vi "TARGET.vi"() -> ()   [LabVIEW 2018]
uses:
  <vilib>/Platform/TimedLoop/XDataNode/timing_clust.ctl
  <vilib>/Platform/TimedLoop/XDataNode/nitl_modes.ctl
  <vilib>/Platform/TimedLoop/XDataNode/wakeup.ctl
  <vilib>/rvi/eio/common/nirviEmuTemplateMethod_errors.vi
  <vilib>/rvi/Emulation/niFpgaGetClockAttributes.vi
  <vilib>/rvi/Emulation/niFpgaSctlEmulationGetInTimedLoop.vi
  <vilib>/rvi/Emulation/niFpgaEmulationReportErrorSimple.vi
  <vilib>/rvi/Emulation/niFpgaProcessEmulError.vi
  <vilib>/rvi/Emulation/niFpgaCriticalErrorInLSC.vi
  <vilib>/rvi/DataTransferAndStorage/Container/Common/niFpgaContainerGetUniqueNameForEmu.vi
  <vilib>/rvi/Memory/Memory_Emulation/niFpgaMemoryFastEmulationDramWriteAndRequestData.vi
  <vilib>/rvi/Memory/Memory_Emulation/niFpgaMemoryEmulationDramWriteAndRequestData.vi
  <vilib>/rvi/Memory/Memory_Emulation/niFpgaMemoryEmulationDramWriteAndRequestDataApplyByteEnables.vi
  <vilib>/rvi/interface/RandomDataEmulation/niFpgaRandomDataHandleErrors.vi
  <vilib>/eio/EIONode/EIONode.xnode
  <vilib>/Platform/TimedLoop/XDataNode/XDataNode.xnode
  <vilib>/rvi/DataTransferAndStorage/Container/XNode/niFpgaContainer.xnode
  <vilib>/rvi/Memory/Memory_Emulation/niFpgaMemoryEmulationDramRetrieveData.vi
  <vilib>/rvi/interface/RandomDataEmulation/nirviRandomDataFpgaReadWriteTemplate.vi
  <vilib>/Platform/TimedLoop/XDataNode/XDNodeRunTimeDep.lvlib
panel:
  in  "17850?":u16=17850
  in  "SUB2":u16=750
  in  "SUB1":u16=550
  in  "Номер SUB":u16=250
  in  "P4B_2@":u16=1700
  in  "P4B_1@":u16=1100
  in  "P4B_2@@":u16=2600
  in  "P4B_1@@":u16=2000
  in  "P1B_2_2":u16=2000
  in  "P1B_2_1":u16=1700
  in  "P1B_1_2":u16=250
  in  "P1B_1_1":u16=50
  in  "P1B_1_2@":u16=2500
  in  "P1B_1_1@":u16=1000
  in  "P4B_2":u16=350
  in  "P4B_1":u16=150
  in  "P3B_2":u16=245
  in  "P3B_1":u16=55
  in  "P3B_2@":u16=2500
  in  "P3B_1@":u16=1000
  in  "P2B_2@":u16=2600
  in  "P2B_1@":u16=1100
  in  "P2B_1":u16=155
  in  "P2B_2":u16=345
  in  "0":u16
  in  "CDS1_1":u8=3
  in  "CDS1_2":u8=5
  in  "CDS2_1":u8=6
  in  "CDS2_2":u8=10
  in  "ADC_1":u8=3
  in  "ADC_2":u8=9
  in  "17846?":u16=17846
  in  "789?":u16=789
  in  "17860?":u16=17860
  in  "P5_1":u8
  in  "P5_2":u8=6
  in  "P6_1":u8
  in  "P6_2":u8=6
  in  "P7_1":u8
  in  "P7_2":u8=2
  in  "P_end":u8=10
  in  "С_1265?":u16=1265
  in  "HIGH":u8=6
  in  "LOW":u8=1
  out "Элем.":u32
  out "Данные":u8
  in  "Направление бит":bool
  in  "Между кадрами":u16 caption="Между кадрами, мс"
  in  "А(T)/А+В(F)":bool=TRUE
  in  "Кадр в память":bool
  in  "Кадр на ПК":bool
  in  "Нач_адр":u32
  in  "1":u8=1
  in  "2":u8=2
  in  "Кон_адр":u32=16384
  out "Записали FIFO":bool
  in  "Линейки":bool
  in  "Command array":bool[](array[boolean])=[FALSE, FALSE, FALSE, FALSE, FALSE, FALSE, FALSE, FALSE, FALSE, FALSE, FALSE, FALSE, FALSE, FALSE, FALSE, FALSE, FALSE]
  in  "Read(T)/Write(F)":bool
  in  "Enum":T1(ring)=enum."GREEN PGA"
  in  "Write Data":bool[](array[boolean])=[FALSE, FALSE, FALSE, FALSE, FALSE, FALSE, FALSE, FALSE, FALSE]
  out "READ":bool[](array[boolean])
  in  "Конфигурация":bool
  in  "Остановка основного цикла":bool
  # "НОРМА"
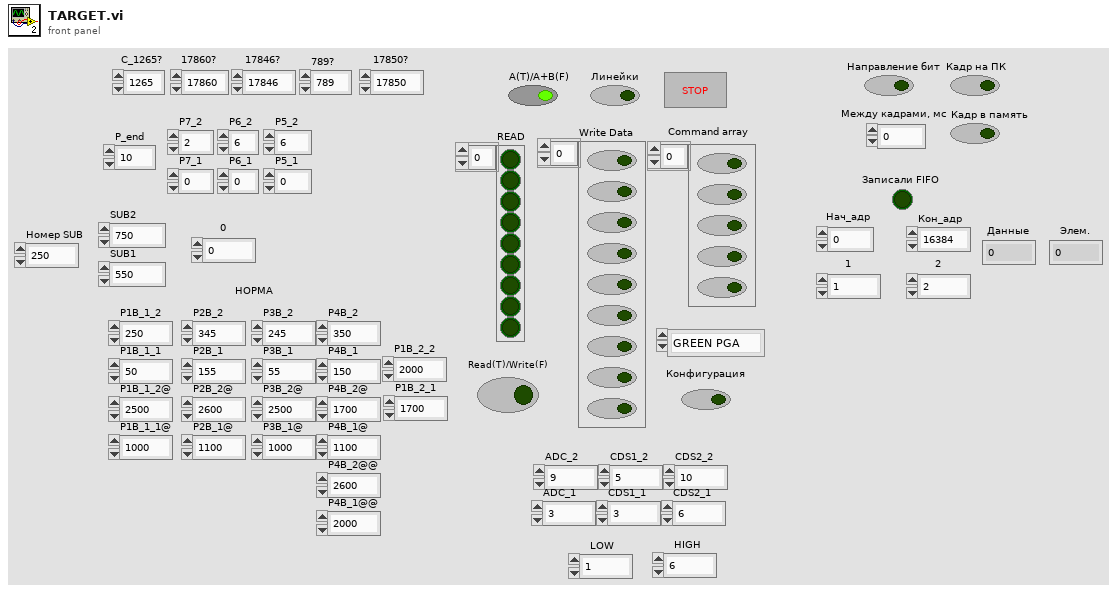
[diagram p1: front panel]
types:
  T1 = enum16{"Configuration", "MUX", "RED PGA", "GREEN PGA", "BLUE PGA", "RED OFF", "GREEN OFF", "BLUE OFF"}
  T2 = typedef "XDNodeRunTimeDep.lvlib/timing_clust.ctl" = cluster{"Expected End [f-1]":u64, "Actual End [f-1]":u64, "Finished Late? [f-1]":bool, "Expected End [i-1]":u64, "Actual End [i-1]":u64, "Finished Late? [i-1]":bool, "Expected Start [i]":u64, "Actual Start [i]":u64, "Expected Start [f]":u64, "Actual Start [f]":u64, "Source Name":string, "Structure Name":string, "Period":i64, "Deadline":i64, "Offset":i64, "Start":i64, "Priority":i32, "Timeout":i32, "Mode":T3, "Wakeup Reason":T4, "Error":errorcluster, "Source Type":string, "Secondary Source Type":string, "Global End Time":u64, "Global Start Time":u64, "Frame Duration":u64, "Iteration Duration":u64, "Assigned CPU":i32, "I/O Scan Engine Mode":u32}
  T3 = typedef "XDNodeRunTimeDep.lvlib/nitl_modes.ctl" = enum32{"No Change", "Process missed periods, maintain original phase", "Discard missed periods, maintain original phase", "Process missed periods, ignore original phase", "Discard missed periods, ignore original phase"}
  T4 = typedef "XDNodeRunTimeDep.lvlib/wakeup.ctl" = enum32{"Normal", "Aborted", "Asynchronous wakeup", "Timing source error", "Timed loop error", "Timeout"}
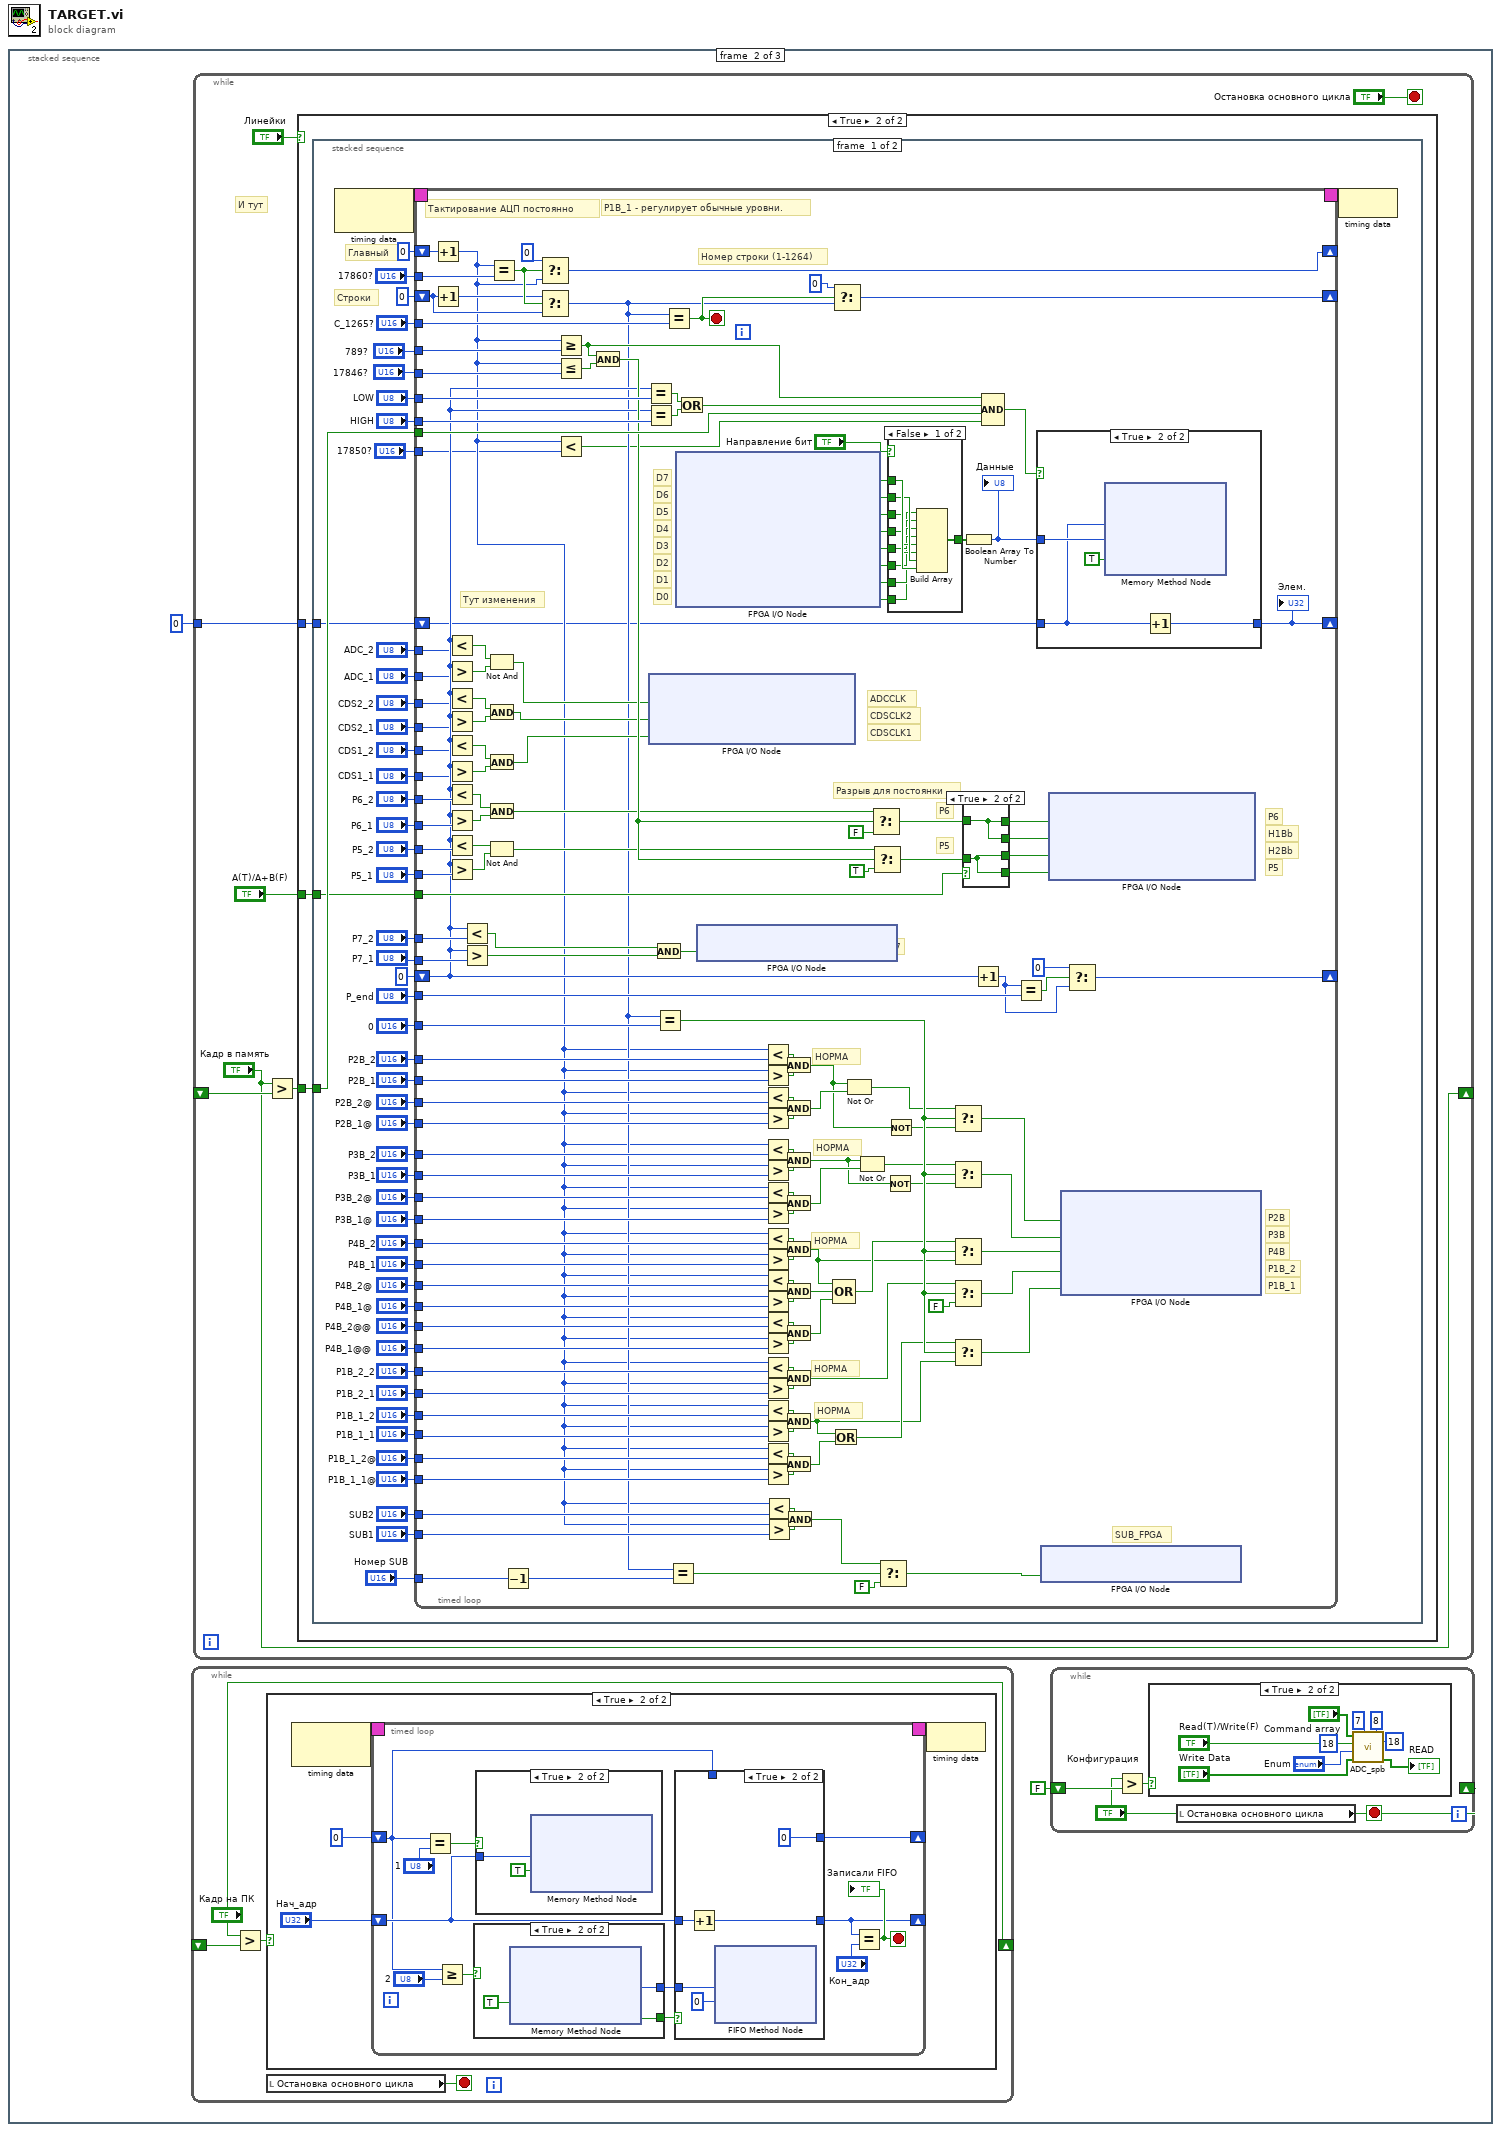
[diagram p0: block diagram]
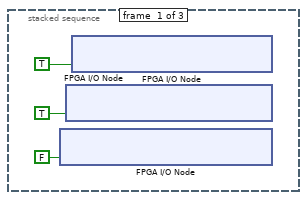
[diagram p2: hidden frame]
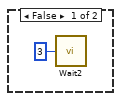
[diagram p3: hidden frame]
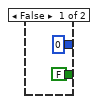
[diagram p4: hidden frame]
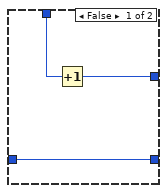
[diagram p6: hidden frame]
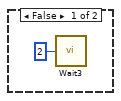
[diagram p7: hidden frame]
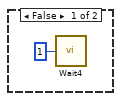
[diagram p8: hidden frame]
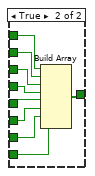
[diagram p10: hidden frame]
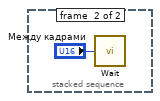
[diagram p12: hidden frame]
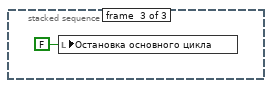
[diagram p13: hidden frame]
diagram:
  n1 = stacked-sequence {
    frame #0 {
      n2 = xnode "FPGA I/O Node"("IO Module\\DDCA_DIO16-23_WE"=FALSE) -> ()  [unwired: 1 in, 1 out]
      n3 = xnode "FPGA I/O Node"("IO Module\\DDCA_DIO8-15_WE"=TRUE) -> ()  [unwired: 1 in, 1 out]
      n4 = xnode "FPGA I/O Node"("IO Module\\DDCA_DIO0-7_WE"=TRUE) -> ()  [unwired: 1 in, 1 out]
    }
    frame #1 {
      n5 = while {
        shift-right: ["Кадр на ПК"] -> _
        shift-left: _ -> [w7]
        stop <- w9 stop-if-true
        n6 = Greater?(x="Кадр на ПК", y=w7) -> (0:w8:bool)
        n7 = case shown="True" w8 {
          frame False {
            n8 = call "Wait2"("Count(Ticks)"=u8 3) -> ()  [unwired: 1 out]
          }
          frame True {
            n9 = node-c288() -> (w14:T2)  [unwired: 1 in]
            n10 = timed-loop {
              shift-right: [w25] -> _
              shift-left: "Нач_адр" -> [w19]
              timing: w14 -> [_]
              timing-out: [_] -> w13
              shift-right: [w16] -> _
              shift-left: u8 0 -> [w17]
              stop <- w26 stop-if-true
              n11 = Equal?(x=w17, y="1") -> (x = y?=w23:bool)
              n12 = Greater Or Equal?(x=w17, y="2") -> (x >= y?=w20:bool)
              n13 = case shown="True" w20 {
                tunnel: [u8 0 ("Data") w31] -> w24
                tunnel: [FALSE ("Output Valid") w30] -> w18
                frame False {
                }
                frame True {
                  n14 = xnode ("Memory Method Node")("Ready for Output"=TRUE ("Ready For Output")) -> ("Data"=w31:u8, "Output Valid"=w30:bool)  [unwired: 1 in, 1 out]
                }
              }
              n15 = case shown="True" w23 {
                tunnel: w19 -> [_ w32]
                frame False {
                }
                frame True {
                  n16 = xnode ("Memory Method Node")("Address"=w32, "Input Valid"=TRUE) -> ()  [unwired: 1 in, 2 out]
                }
              }
              n17 = case shown="True" w18 {
                tunnel: [w34 w41] -> w25
                tunnel: w24 -> [_ w38]
                tunnel: w19 -> [w34 w40]
                tunnel: w17 -> [w36 _]
                tunnel: [w35 u8 0] -> w16
                frame False {
                  n18 = Increment(x=w36) -> (x+1=w35:u8)
                }
                frame True {
                  n19 = Increment(x=w40) -> (x+1=w41:u32)
                  n20 = xnode ("FIFO Method Node")("Element"=w38, "Timeout"=0) -> ()  [unwired: 1 in, 2 out]
                }
              }
              n21 = Equal?(x=w25, y="Кон_адр") -> (x = y?=w26:bool)
              "Записали FIFO" <- w26
            }
            n22 = node-c288(w13) -> ()
          }
        }
        n23 = local read "Остановка основного цикла"() -> (w9:bool)
      }
      n24 = while {
        shift-right: ["Кадр в память"] -> _
        shift-left: _ -> [w65]
        tunnel: u32 0 -> [w60]
        stop <- "Остановка основного цикла" stop-if-true
        # "И тут"
        n25 = Greater?(x="Кадр в память", y=w65) -> (0:w64:bool)
        n26 = case shown="True" "Линейки" {
          tunnel: w64 -> [_ w70]
          tunnel: "А(T)/А+В(F)" -> [_ w69]
          tunnel: w60 -> [_ w68]
          frame False {
            n27 = call "Wait4"("Count(Ticks)"=u8 1) -> ()  [unwired: 1 out]
          }
          frame True {
            n28 = stacked-sequence {
              tunnel: w70 -> [w122 _]
              tunnel: w69 -> [w121 _]
              tunnel: w68 -> [w71 _]
              frame #0 {
                # "Строки"
                # "Главный"
                n29 = node-c288() -> (w120:T2)  [unwired: 1 in]
                n30 = timed-loop {
                  timing: w120 -> [_]
                  timing-out: [_] -> w119
                  tunnel: w122 -> [w266]
                  tunnel: w121 -> [w281]
                  tunnel: "LOW" -> [w262]
                  tunnel: "HIGH" -> [w261]
                  tunnel: "С_1265?" -> [w235]
                  shift-right: [w249] -> _
                  shift-left: u8 0 -> [w220]
                  tunnel: "P_end" -> [w253]
                  tunnel: "P7_2" -> [w252]
                  tunnel: "P7_1" -> [w245]
                  tunnel: "P6_2" -> [w247]
                  tunnel: "P6_1" -> [w248]
                  tunnel: "P5_2" -> [w244]
                  tunnel: "P5_1" -> [w243]
                  shift-right: [w239] -> _
                  shift-left: u16 0 -> [w242]
                  tunnel: "17860?" -> [w241]
                  shift-right: [w136] -> _
                  shift-left: u16 0 -> [w236]
                  tunnel: "789?" -> [w234]
                  tunnel: "17846?" -> [w231]
                  tunnel: "ADC_2" -> [w219]
                  tunnel: "ADC_1" -> [w218]
                  tunnel: "CDS2_2" -> [w217]
                  tunnel: "CDS2_1" -> [w216]
                  tunnel: "CDS1_2" -> [w215]
                  tunnel: "CDS1_1" -> [w214]
                  tunnel: "0" -> [w204]
                  tunnel: "Номер SUB" -> [w130]
                  tunnel: "P2B_2" -> [w164]
                  tunnel: "P2B_1" -> [w163]
                  tunnel: "P2B_2@" -> [w162]
                  tunnel: "P2B_1@" -> [w161]
                  tunnel: "P3B_2" -> [w160]
                  tunnel: "P3B_1" -> [w159]
                  tunnel: "P3B_2@" -> [w158]
                  tunnel: "P3B_1@" -> [w157]
                  tunnel: "P4B_2" -> [w156]
                  tunnel: "P4B_1" -> [w155]
                  tunnel: "P4B_2@" -> [w154]
                  tunnel: "P4B_1@" -> [w153]
                  tunnel: "P4B_2@@" -> [w152]
                  tunnel: "P4B_1@@" -> [w151]
                  tunnel: "P1B_2_2" -> [w150]
                  tunnel: "P1B_2_1" -> [w149]
                  tunnel: "P1B_1_2" -> [w148]
                  tunnel: "P1B_1_1" -> [w147]
                  tunnel: "P1B_1_2@" -> [w146]
                  tunnel: "P1B_1_1@" -> [w145]
                  tunnel: "SUB2" -> [w142]
                  tunnel: "SUB1" -> [w141]
                  tunnel: "17850?" -> [w126]
                  shift-right: [w123] -> _
                  shift-left: w71 -> [w124]
                  stop <- w139 stop-if-true
                  # "Тут изменения"
                  # "SUB_FPGA"
                  # "НОРМА"
                  # "НОРМА"
                  # "НОРМА"
                  # "НОРМА"
                  # "НОРМА"
                  # "P1B_1"
                  # "P1B_2"
                  # "P4B"
                  # "P3B"
                  # "P2B"
                  # "CDSCLK1"
                  # "CDSCLK2"
                  # "ADCCLK"
                  # "Номер строки (1-1264)"
                  # "Разрыв для постоянки"
                  # "P5"
                  # "P6"
                  # "P1B_1 - регулирует обычные уровни."
                  # "P5"
                  # "H2Bb"
                  # "H1Bb"
                  # "P6"
                  # "P7"
                  # "D0"
                  # "D1"
                  # "D2"
                  # "D3"
                  # "D4"
                  # "D5"
                  # "D6"
                  # "D7"
                  # "Тактирование АЦП постоянно"
                  n31 = Increment(x=w242) -> (x+1=w127:u16)
                  n32 = Increment(x=w236) -> (x+1=w237:u16)
                  n33 = Less?(x=w220, y=w219) -> (x < y?=w226:bool)
                  n34 = Greater?(x=w220, y=w218) -> (0:w225:bool)
                  n35 = Less?(x=w220, y=w217) -> (x < y?=w223:bool)
                  n36 = Greater?(x=w220, y=w216) -> (0:w224:bool)
                  n37 = Less?(x=w220, y=w215) -> (x < y?=w222:bool)
                  n38 = Greater?(x=w220, y=w214) -> (0:w221:bool)
                  n39 = Less?(x=w220, y=w247) -> (x < y?=w257:bool)
                  n40 = Greater?(x=w220, y=w248) -> (0:w260:bool)
                  n41 = Less?(x=w220, y=w244) -> (x < y?=w259:bool)
                  n42 = Greater?(x=w220, y=w243) -> (0:w258:bool)
                  n43 = Less?(x=w220, y=w252) -> (x < y?=w255:bool)
                  n44 = Greater?(x=w220, y=w245) -> (0:w254:bool)
                  n45 = Not And(1:w225, 2:w226) -> (0:w207:bool)
                  n46 = And(x=w223, y=w224) -> (x .and. y?=w208:bool)
                  n47 = And(x=w222, y=w221) -> (x .and. y?=w209:bool)
                  n48 = And(x=w257, y=w260) -> (x .and. y?=w213:bool)
                  n49 = Not And(1:w258, 2:w259) -> (0:w212:bool)
                  n50 = Equal?(x=w127, y=w241) -> (x = y?=w238:bool)
                  n51 = Decrement(x=w130) -> (x-1=w129:u16)
                  n52 = Select(t=u16 0, s=w238, f=w127) -> (s? t:f=w239:u16)
                  n53 = Select(t=w237, s=w238, f=w236) -> (s? t:f=w137:u16)
                  n54 = Greater Or Equal?(x=w127, y=w234) -> (x >= y?=w210:bool)
                  n55 = Less Or Equal?(x=w127, y=w231) -> (x <= y?=w230:bool)
                  n56 = Less?(x=w127, y=w126) -> (x < y?=w128:bool)
                  n57 = And(x=w210, y=w230) -> (x .and. y?=w229:bool)
                  n58 = Equal?(x=w220, y=w262) -> (x = y?=w264:bool)
                  n59 = Equal?(x=w220, y=w261) -> (x = y?=w265:bool)
                  n60 = xnode "FPGA I/O Node"("IO Module\\DDCA_DIO9_Write"=w207, "IO Module\\DDCA_DIO10_Write"=w208, "IO Module\\DDCA_DIO11_Write"=w209) -> ()  [unwired: 3 in, 3 out]
                  n61 = And(x=w255, y=w254) -> (x .and. y?=w211:bool)
                  n62 = Equal?(x=w137, y=w204) -> (x = y?=w203:bool)
                  n63 = Equal?(x=w137, y=w235) -> (x = y?=w139:bool)
                  n64 = Equal?(x=w137, y=w129) -> (x = y?=w167:bool)
                  n65 = xnode "FPGA I/O Node"() -> ("IO Module\\DDCA_DIO16_Read"=w276:bool, "IO Module\\DDCA_DIO17_Read"=w275:bool, "IO Module\\DDCA_DIO18_Read"=w269:bool, "IO Module\\DDCA_DIO19_Read"=w270:bool, "IO Module\\DDCA_DIO20_Read"=w271:bool, "IO Module\\DDCA_DIO21_Read"=w272:bool, "IO Module\\DDCA_DIO22_Read"=w273:bool, "IO Module\\DDCA_DIO23_Read"=w274:bool)  [unwired: 8 in, 8 out]
                  n66 = Or(x=w264, y=w265) -> (x .or. y?=w263:bool)
                  n67 = xnode "FPGA I/O Node"("IO Module\\DDCA_DIO0_Write"=w211) -> ()  [unwired: 1 in, 1 out]
                  n68 = Less?(x=w127, y=w164) -> (x < y?=w205:bool)
                  n69 = Greater?(x=w127, y=w163) -> (0:w206:bool)
                  n70 = Less?(x=w127, y=w162) -> (x < y?=w196:bool)
                  n71 = Greater?(x=w127, y=w161) -> (0:w195:bool)
                  n72 = Less?(x=w127, y=w160) -> (x < y?=w192:bool)
                  n73 = Greater?(x=w127, y=w159) -> (0:w191:bool)
                  n74 = Less?(x=w127, y=w158) -> (x < y?=w193:bool)
                  n75 = Greater?(x=w127, y=w157) -> (0:w194:bool)
                  n76 = Less?(x=w127, y=w156) -> (x < y?=w189:bool)
                  n77 = Greater?(x=w127, y=w155) -> (0:w190:bool)
                  n78 = Less?(x=w127, y=w154) -> (x < y?=w188:bool)
                  n79 = Greater?(x=w127, y=w153) -> (0:w187:bool)
                  n80 = Less?(x=w127, y=w152) -> (x < y?=w184:bool)
                  n81 = Greater?(x=w127, y=w151) -> (0:w183:bool)
                  n82 = Less?(x=w127, y=w150) -> (x < y?=w185:bool)
                  n83 = Greater?(x=w127, y=w149) -> (0:w186:bool)
                  n84 = Less?(x=w127, y=w148) -> (x < y?=w182:bool)
                  n85 = Greater?(x=w127, y=w147) -> (0:w181:bool)
                  n86 = Less?(x=w127, y=w146) -> (x < y?=w171:bool)
                  n87 = Greater?(x=w127, y=w145) -> (0:w172:bool)
                  n88 = Less?(x=w127, y=w142) -> (x < y?=w144:bool)
                  n89 = Greater?(x=w127, y=w141) -> (0:w143:bool)
                  n90 = And(x=w205, y=w206) -> (x .and. y?=w133:bool)
                  n91 = And(x=w196, y=w195) -> (x .and. y?=w180:bool)
                  n92 = And(x=w192, y=w191) -> (x .and. y?=w132:bool)
                  n93 = And(x=w193, y=w194) -> (x .and. y?=w179:bool)
                  n94 = And(x=w189, y=w190) -> (x .and. y?=w174:bool)
                  n95 = And(x=w188, y=w187) -> (x .and. y?=w177:bool)
                  n96 = And(x=w184, y=w183) -> (x .and. y?=w176:bool)
                  n97 = And(x=w185, y=w186) -> (x .and. y?=w173:bool)
                  n98 = And(x=w182, y=w181) -> (x .and. y?=w168:bool)
                  n99 = And(x=w171, y=w172) -> (x .and. y?=w170:bool)
                  n100 = And(x=w144, y=w143) -> (x .and. y?=w140:bool)
                  n101 = Or(x=w168, y=w170) -> (x .or. y?=w169:bool)
                  n102 = Select(t=u16 0, s=w139, f=w137) -> (s? t:f=w136:u16)
                  n103 = Compound Arithmetic op=OR(w174, w177, w176) -> (w175:bool)
                  n104 = Not Or(1:w180, 2:w133) -> (0:w135:bool)
                  n105 = Not Or(1:w179, 2:w132) -> (0:w178:bool)
                  n106 = Select(t=w213, s=w229, f=FALSE ("t")) -> (s? t:f=w233:bool)
                  n107 = Select(t=w212, s=w229, f=TRUE ("t")) -> (s? t:f=w232:bool)
                  n108 = Select(t=w140, s=w167, f=FALSE) -> (s? t:f=w165:bool)
                  n109 = Not(x=w132) -> (.not. x?=w131:bool)
                  n110 = Not(x=w133) -> (.not. x?=w134:bool)
                  n111 = case shown="False" "Направление бит" {
                    tunnel: w276 -> [w294 w304]
                    tunnel: w275 -> [w293 w303]
                    tunnel: w269 -> [w292 w302]
                    tunnel: w270 -> [w291 w301]
                    tunnel: w271 -> [w290 w300]
                    tunnel: w272 -> [w289 w299]
                    tunnel: w273 -> [w288 w298]
                    tunnel: w274 -> [w287 w297]
                    tunnel: [w295 w296] -> w268
                    frame False {
                      n112 = Build Array(w287, w288, w289, w290, w291, w292, w293, w294) -> (w295:bool[])
                    }
                    frame True {
                      n113 = Build Array(w304, w303, w302, w301, w300, w299, w298, w297) -> (w296:bool[])
                    }
                  }
                  n114 = Select(t=w135, s=w203, f=w134) -> (s? t:f=w202:bool)
                  n115 = Select(t=w178, s=w203, f=w131) -> (s? t:f=w201:bool)
                  n116 = Select(t=w175, s=w203, f=w174) -> (s? t:f=w200:bool)
                  n117 = Select(t=w173, s=w203, f=FALSE) -> (s? t:f=w199:bool)
                  n118 = Select(t=w169, s=w203, f=w168) -> (s? t:f=w198:bool)
                  n119 = case shown="True" w281 {
                    tunnel: w233 -> [w306 w308]
                    tunnel: w232 -> [w305 w307]
                    tunnel: [w305 w308] -> w280
                    tunnel: [w306 w307] -> w279
                    tunnel: [w306 w308] -> w278
                    tunnel: [w305 w307] -> w277
                    frame False {
                    }
                    frame True {
                    }
                  }
                  n120 = Boolean Array To Number(Boolean array=w268) -> (number=w267:u8)
                  "Данные" <- w267
                  n121 = Increment(x=w220) -> (x+1=w246:u8)
                  n122 = Compound Arithmetic op=AND(w210, w263, w266, w128) -> (w125:bool)
                  n123 = Equal?(x=w246, y=w253) -> (x = y?=w251:bool)
                  n124 = case shown="True" w125 {
                    tunnel: w267 -> [_ w286]
                    tunnel: w124 -> [w282 w284]
                    tunnel: [w282 w283] -> w123
                    frame False {
                    }
                    frame True {
                      n125 = xnode ("Memory Method Node")("Address"=w284, "Data"=w286, "Input Valid"=TRUE) -> ()  [unwired: 1 in, 2 out]
                      n126 = Increment(x=w284) -> (x+1=w283:u32)
                    }
                  }
                  "Элем." <- w123
                  n127 = xnode "FPGA I/O Node"("IO Module\\DDCA_DIO1_Write"=w165) -> ()  [unwired: 1 in, 1 out]
                  n128 = xnode "FPGA I/O Node"("IO Module\\DDCA_DIO12_Write"=w278, "IO Module\\DDCA_DIO13_Write"=w280, "IO Module\\DDCA_DIO14_Write"=w279, "IO Module\\DDCA_DIO15_Write"=w277) -> ()  [unwired: 4 in, 4 out]
                  n129 = xnode "FPGA I/O Node"("IO Module\\DDCA_DIO2_Write"=w202, "IO Module\\DDCA_DIO3_Write"=w201, "IO Module\\DDCA_DIO4_Write"=w200, "IO Module\\DDCA_DIO5_Write"=w199, "IO Module\\DDCA_DIO6_Write"=w198) -> ()  [unwired: 5 in, 5 out]
                  n130 = Select(t=u8 0, s=w251, f=w246) -> (s? t:f=w249:u8)
                }
                n131 = node-c288(w119) -> ()
              }
              frame #1 {
                n132 = call "Wait"("Count(mSec)"="Между кадрами") -> ()  [unwired: 1 out]
              }
            }
          }
        }
      }
      n133 = while {
        shift-right: ["Конфигурация"] -> _
        shift-left: FALSE ("Конфигурация") -> [w48]
        stop <- w49 stop-if-true
        n134 = Greater?(x="Конфигурация", y=w48) -> (0:w46:bool)
        n135 = case shown="True" w46 {
          frame False {
            n136 = call "Wait3"("Count(Ticks)"=u8 2) -> ()  [unwired: 1 out]
          }
          frame True {
            n137 = call "ADC_spb.vi"(1:"18_1"=i8 18 ("18_1"), 2:"18_1"=i8 18 ("18_1"), "8"=i8 8, "7"=i8 7, "Write Data"="Write Data", "Enum"="Enum", "Read(T)/Write(F)"="Read(T)/Write(F)", "Command array"="Command array") -> ("READ"=→"READ":bool[])
          }
        }
        n138 = local read "Остановка основного цикла"() -> (w49:bool)
      }
    }
    frame #2 {
      n139 = local write "Остановка основного цикла"(FALSE ("Остановка основного цикла")) -> ()
    }
  }
